vi "GetType.vi"(8 "error in (no error)":errorcluster, 11 "Abort Msg":refnum<class "Abort Msg.lvclass">) -> (0 "error out":errorcluster, 2 "Data Sample":variant, 3 "Abort Msg":refnum<class "Abort Msg.lvclass">)   [LabVIEW 2015, in "CS++DMM.lvlib" / "Abort Msg.lvclass"]
uses:
  Abort Msg.lvclass
  Abort Msg.lvclass/Abort Msg.ctl
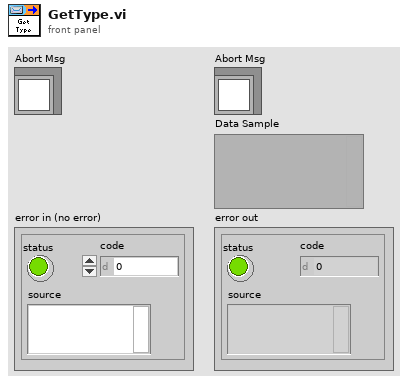
[diagram p1: front panel]
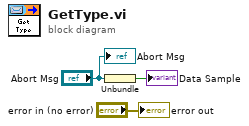
[diagram p0: block diagram]
diagram:
  n1 = Unbundle("Abort Msg") -> (→"Data Sample":bool)
  "error out" <- "error in (no error)"
  "Abort Msg" <- "Abort Msg"
